vi "AvoidCarla.vi"(8 "Events.Touch":bool, 11 "command\nenum":T1) -> (2 "Avoid":bool)   [LabVIEW 2016]
uses:
  Command Enum.ctl
panel:
  out "State":enum16{"Avoid", "Normal", "First kick"}(ring)
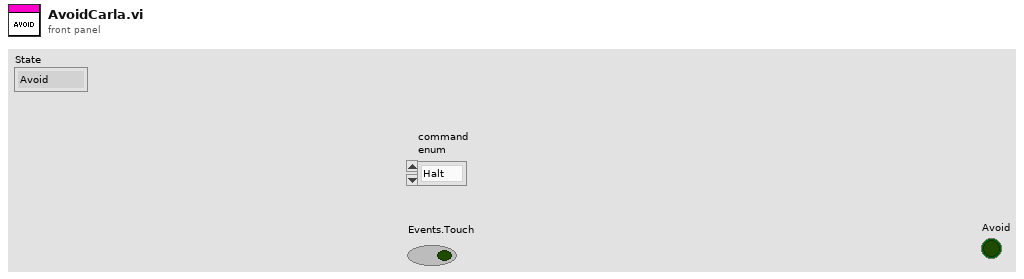
[diagram p1: front panel]
types:
  T1 = typedef "Command Enum.ctl" = enum16{"Halt", "Stop", "Force Start", "PKA Normal Start", "Prepare Kickoff Ally", "PKE Normal Start", "Prepare Kickoff Enemy", "Prepare Penalty Ally", "PPA Normal Start", "Prepare Penalty Enemy", "PPE Normal Start", "Direct Free Enemy", "Direct Free Ally", "Indirect Free Enemy", "Indirect Free Ally", "Timeout Enemy", "Timeout Ally", "Goal Enemy", "Goal Ally", "Ball Placement Enemy", "Ball Placement Ally", "None"}
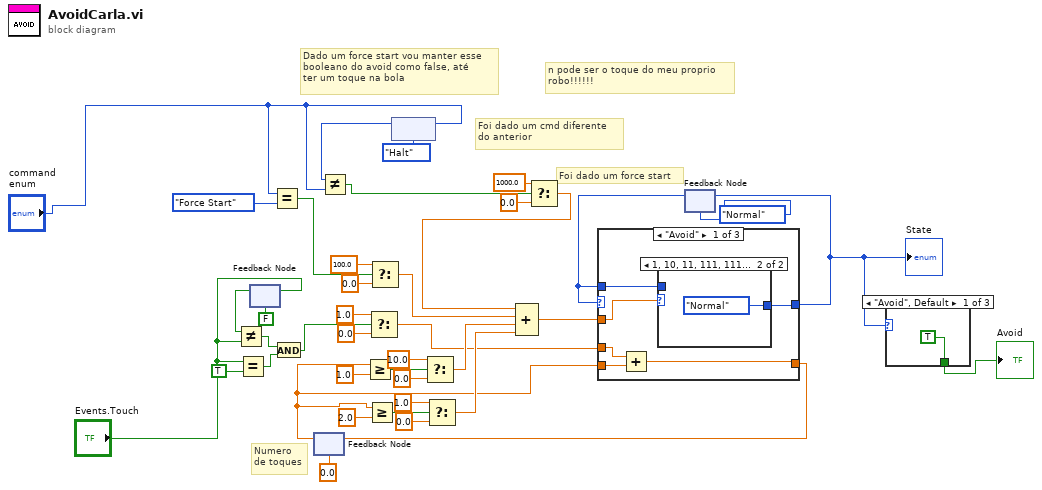
[diagram p0: block diagram]
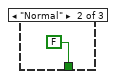
[diagram p2: hidden frame]
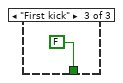
[diagram p3: hidden frame]
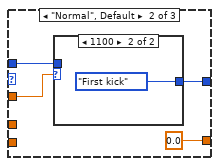
[diagram p5: hidden frame]
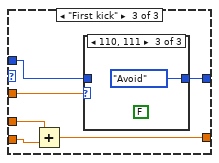
[diagram p7: hidden frame]
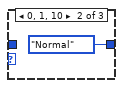
[diagram p9: hidden frame]
diagram:
  # "n pode ser o toque do meu proprio\nrobo!!!!!!"
  # "Dado um force start vou manter esse\nbooleano do avoid como false, até\nter um toque na bola"
  # "Numero\nde toques"
  # "Foi dado um force start"
  # "Foi dado um cmd diferente\ndo anterior"
  n1 = Equal?(x="Events.Touch", y=TRUE) -> (x = y?=w27:bool)
  n2 = feedback #1(FALSE ("Touch")) -> (w32:bool)
  n3 = Not Equal?(x=w32, y="Events.Touch") -> (x != y?=w28:bool)
  n4 = feedback-in #1("Events.Touch") -> ()
  n5 = Equal?(x="command\nenum", y=Command_Enum."Force Start" ("command\nenum")) -> (x = y?=w29:bool)
  n6 = And(x=w28, y=w27) -> (x .and. y?=w23:bool)
  n7 = feedback #2(0.0) -> (w8:dbl)
  n8 = Greater Or Equal?(x=w8, y=1.0) -> (x >= y?=w11:bool)
  n9 = Greater Or Equal?(x=w8, y=2.0) -> (x >= y?=w10:bool)
  n10 = Select(t=1.0, s=w23, f=0.0) -> (s? t:f=w9:dbl)
  n11 = Select(t=100.0, s=w29, f=0.0) -> (s? t:f=w37:dbl)
  n12 = feedback #3(Command_Enum."Halt" ("command\nenum")) -> (w26:T1)
  n13 = Not Equal?(x=w26, y="command\nenum") -> (x != y?=w4:bool)
  n14 = feedback-in #3("command\nenum") -> ()
  n15 = Select(t=10.0, s=w11, f=0.0) -> (s? t:f=w15:dbl)
  n16 = Select(t=1.0, s=w10, f=0.0) -> (s? t:f=w12:dbl)
  n17 = Select(t=1000.0, s=w4, f=0.0) -> (s? t:f=w38:dbl)
  n18 = Compound Arithmetic op=ADD(w38, w37, w15, w12) -> (w20:dbl)
  n19 = feedback #4(enum16{"Avoid", "Normal", "First kick"}."Normal" ("State")) -> (w19:enum16{"Avoid", "Normal", "First kick"})
  n20 = case shown="\"Avoid\"" w19 {
    tunnel: w20 -> [w46 w52 w60]
    tunnel: [w45 w51 w59] -> w6
    tunnel: w19 -> [w44 w50 w58]
    tunnel: w9 -> [w42 _ w57]
    tunnel: w8 -> [w43 _ w56]
    tunnel: [w41 0.0 w55] -> w7
    frame "Avoid" {
      n21 = Add(x=w42, y=w43) -> (x+y=w41:dbl)
      n22 = case shown="1, 10, 11, 111, 1111" w46 {
        tunnel: [w47 enum16{"Avoid", "Normal", "First kick"}."Normal" ("State")] -> w45
        tunnel: w44 -> [w47 _]
        frame Default {
        }
        frame 1, 10, 11, 111, 1111 {
        }
      }
    }
    frame "Normal", Default {
      n23 = case shown="1100" w52 {
        tunnel: [w53 enum16{"Avoid", "Normal", "First kick"}."First kick" ("State")] -> w51
        tunnel: w50 -> [w53 _]
        frame Default {
        }
        frame 1100 {
        }
      }
    }
    frame "First kick" {
      n24 = Add(x=w57, y=w56) -> (x+y=w55:dbl)
      n25 = case shown="110, 111" w60 {
        tunnel: [w61 enum16{"Avoid", "Normal", "First kick"}."Normal" ("State") enum16{"Avoid", "Normal", "First kick"}."Avoid" ("State")] -> w59
        tunnel: w58 -> [w61 _ _]
        frame Default {
        }
        frame 0, 1, 10 {
        }
        frame 110, 111 {
          (unwired) FALSE
        }
      }
    }
  }
  "State" <- w6
  n26 = feedback-in #2(w7) -> ()
  n27 = feedback-in #4(w6) -> ()
  n28 = case shown="\"Avoid\", Default" w6 {
    tunnel: [TRUE FALSE FALSE] -> w2
    frame "Avoid", Default {
    }
    frame "Normal" {
    }
    frame "First kick" {
    }
  }
  "Avoid" <- w2
